vi "ConfigureClk.vi"(8 "error in (no error)":errorcluster, 10 "ClkName":string, 11 "NiPxi6683H in":refnum<class "NiPxi6683H.lvclass">) -> (0 "error out":errorcluster, 3 "NiPxi6683H out":refnum<class "NiPxi6683H.lvclass">)   [LabVIEW 2014, in "SyncPlugins.lvlib" / "NiPxi6683H.lvclass"]
uses:
  NiPxi6683H.lvclass
  NiPxi6683H.lvclass/NiPxi6683H.ctl
  NiPxi6682/NiPxi6682.lvclass/NiPxi6682.ctl
  NiPxi6682/Accessors/Read NiSyncHandle.vi
  NiPxi6682/Accessors/Write NiSyncHandle.vi
  Accessors/Write Clocks.vi
  Accessors/Read Clocks.vi
  <vilib>/Utility/error.llb/Error Cluster From Error Code.vi
  <instrlib>/niSync/niSync.llb/niSync Create Clock (Frequency).vi
  <vilib>/ErrorRing/Error Ring.xnode
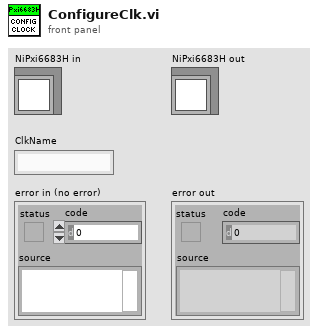
[diagram p1: front panel]
types:
  T1 = typedef "SyncPlugins.lvlib/PXI_MultiTrig.lvclass/clClocks.ctl" = cluster{"Name":string, "RefClk":string, "ClkTerminal":string, "Frequency":dbl, "DutyCycle":dbl, "ClkType":string, "Initiated":bool, "TrigTime":bool}
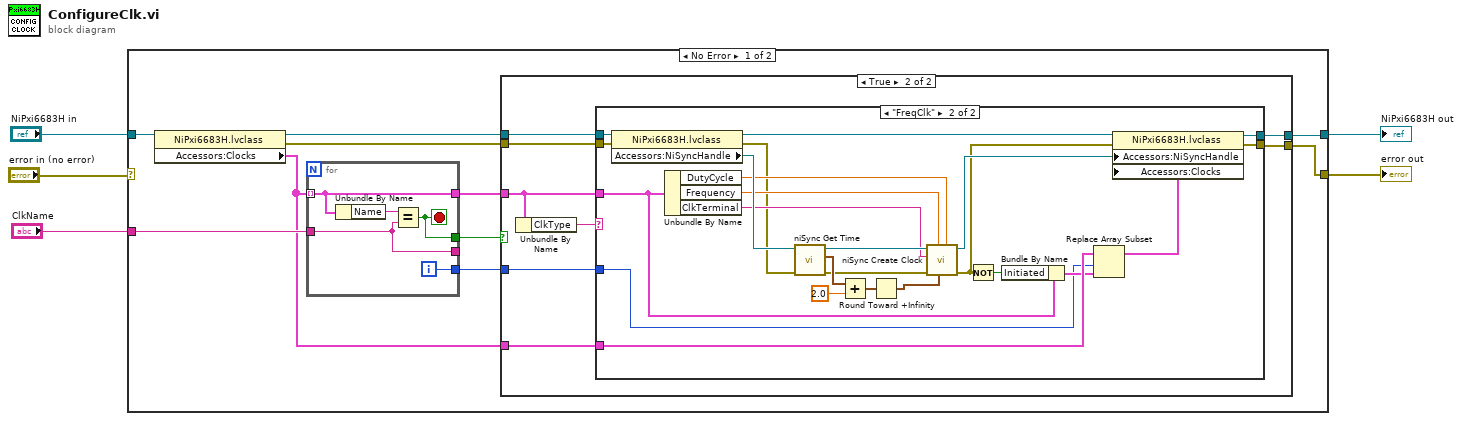
[diagram p0: block diagram]
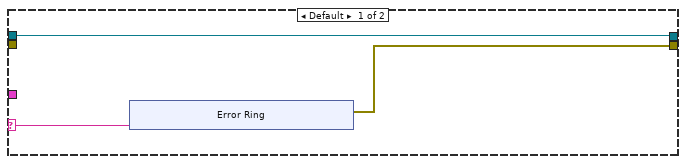
[diagram p3: hidden frame]
diagram:
  n1 = case shown="No Error" "error in (no error)" {
    selector: "error in (no error)" -> [_ w65]
    tunnel: "NiPxi6683H in" -> [w15 w66]
    tunnel: [w7 w66] -> w3
    tunnel: [w6 w65] -> w2
    tunnel: "ClkName" -> [w14 _]
    frame No Error {
      n2 = property class="NiPxi6683H.lvclass"(reference=w15) -> (reference out=w12:refnum<class "NiPxi6683H.lvclass">, error out=w11:errorcluster, "Accessors:Clocks"=w8:T1[])  [unwired: 1 in]
      n3 = for {
        tunnel: w8 -> [w63] mode=indexing
        tunnel: w14 -> [w61]
        tunnel: [w63] -> w9
        tunnel: [w62] -> w10
        tunnel: [w61] -> _
        tunnel: [w60] -> w13
        i -> [w60]
        stop <- w62 stop-if-true
        n4 = Unbundle By Name(w63) -> ("Name"=w64:string)
        n5 = Equal?(x=w64, y=w61) -> (x = y?=w62:bool)
      }
      n6 = case shown="True" w10 {
        tunnel: w13 -> [_ w22]
        tunnel: w12 -> [w17 w25]
        tunnel: w11 -> [w16 w24]
        tunnel: w9 -> [_ w19]
        tunnel: w8 -> [_ w23]
        tunnel: [w17 w21] -> w7
        tunnel: [w16 w20] -> w6
        frame False {
        }
        frame True {
          n7 = Unbundle By Name(w19) -> ("ClkType"=w18:string)
          n8 = case shown="\"FreqClk\"" w18 {
            selector: w18 -> [w28 _]
            tunnel: w25 -> [w27 w59]
            tunnel: w24 -> [_ w58]
            tunnel: w19 -> [_ w48]
            tunnel: w23 -> [_ w46]
            tunnel: w22 -> [_ w44]
            tunnel: [w27 w38] -> w21
            tunnel: [w26 w37] -> w20
            frame Default {
              n9 = xnode "Error Ring"("parameter 0"=w28) -> ("error out"=w26:errorcluster)
            }
            frame "FreqClk" {
              n10 = property class="NiPxi6683H.lvclass"(reference=w59, error in=w58) -> (reference out=w43:refnum<class "NiPxi6683H.lvclass">, error out=w42:errorcluster, "Accessors:NiSyncHandle"=w57:refnum<k15>)
              n11 = Unbundle By Name(w48) -> ("DutyCycle"=w51:dbl, "Frequency"=w50:dbl, "ClkTerminal"=w49:string)
              n12 = call <instrlib>:"niSync Get Time.vi"("error in (no error)"=w42, "instrument handle"=w57) -> ("error out"=w54:errorcluster, "time"=w56:timestamp, "instrument handle out"=w52:refnum<k15>)  [unwired: 5 in]
              n13 = Add(x=w56, y=2.0) -> (x+y=w55:timestamp)
              n14 = Round Toward +Infinity(x=w55) -> (ceil(x): smallest int >= x=w53:timestamp)
              n15 = call-poly <instrlib>:"niSync Create Clock.vi"("duty cycle"=w51, "start time"=w53, "frequency"=w50, "error in (no error)"=w54, "terminal"=w49, "instrument handle"=w52) -> ("error out"=w40:errorcluster, "instrument handle out"=w41:refnum<k15>)  [unwired: 2 in, 2 out]
              n16 = Not(x=w40) -> (.not. x?=w47:bool)
              n17 = Bundle By Name(cluster=w48, "Initiated"=w47) -> (w45:T1)
              n18 = Replace Array Subset(array=w46, new element=w45, index=w44) -> (w39:T1[])
              n19 = property class="NiPxi6683H.lvclass"(reference=w43, error in=w40, "Accessors:NiSyncHandle"=w41, "Accessors:Clocks"=w39) -> (reference out=w38:refnum<class "NiPxi6683H.lvclass">, error out=w37:errorcluster)
            }
          }
        }
      }
    }
    frame Error {
    }
  }
  "error out" <- w2
  "NiPxi6683H out" <- w3
